vi "Supervisor Read Client.vi"() -> ()   [LabVIEW 2017]
uses:
  <vilib>/OPCUA/controls/NodeIds.ctl
  <vilib>/OPCUA/controls/NodeId.ctl
  <vilib>/OPCUA/NI OPC UA Client.lvlib
panel:
  in  "error in (no error)":errorcluster
  in  "stop":bool
  out "error out":errorcluster
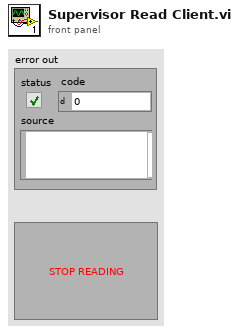
[diagram p1: front panel]
types:
  T1 = cluster{"message mode":enum16{"None", "Sign", "Sign and Encrypt"}, "security":enum16{"Basic256", "Basic128Rsa15"}}
  T2 = typedef "NodeIds.ctl" = T3[]
  T3 = typedef "NodeId.ctl" = string
  T4 = typedef "OPC UA Client Refnum.ctl" = refnum<k21>
  T5 = typedef "Subscription ID.ctl" = u32
  T6 = typedef "Subscription Data Change.ctl" = cluster{"node ID":T3, " value":variant, "timestamp":timestamp, "data type":T7, "status code":T8}
  T7 = typedef "Data Type.ctl" = u16
  T8 = typedef "OPC UA StatusCode.ctl" = u32
  T9 = cluster{"[0]":sgl, "[1]":sgl, "[2]":sgl, "[3]":sgl, "[4]":sgl, "[5]":sgl, "[6]":sgl, "[7]":sgl, "[8]":sgl, "[9]":sgl, "[10]":sgl, "[11]":sgl, "[12]":sgl, "[13]":sgl, "[14]":sgl, "[15]":sgl, "[16]":sgl, "[17]":sgl, "[18]":sgl, "[19]":sgl, "[20]":sgl, "[21]":sgl, "[22]":sgl, "[23]":sgl, "[24]":sgl, "[25]":sgl, "[26]":sgl, "[27]":sgl, "[28]":sgl, "[29]":sgl, "[30]":sgl, "[31]":sgl, "[32]":sgl, "[33]":sgl, "[34]":sgl, "[35]":sgl, "[36]":sgl, "[37]":sgl, "[38]":sgl, "[39]":sgl, "[40]":sgl, "[41]":sgl, "[42]":sgl, "[43]":sgl, "[44]":sgl, "[45]":sgl, "[46]":sgl, "[47]":sgl, "[48]":sgl, "[49]":sgl, "[50]":sgl, "[51]":sgl, "[52]":sgl, "[53]":sgl, "[54]":sgl, "[55]":sgl, "[56]":sgl, "[57]":sgl, "[58]":sgl, "[59]":sgl, "[60]":sgl, "[61]":sgl, "[62]":sgl}
  T10 = cluster{"[0]":sgl, "[1]":sgl, "[2]":sgl, "[3]":sgl, "[4]":sgl, "[5]":sgl, "[6]":sgl, "[7]":sgl, "[8]":sgl, "[9]":sgl}
  T11 = cluster{"[0]":bool, "[1]":bool, "[2]":bool, "[3]":bool, "[4]":bool, "[5]":bool, "[6]":bool}
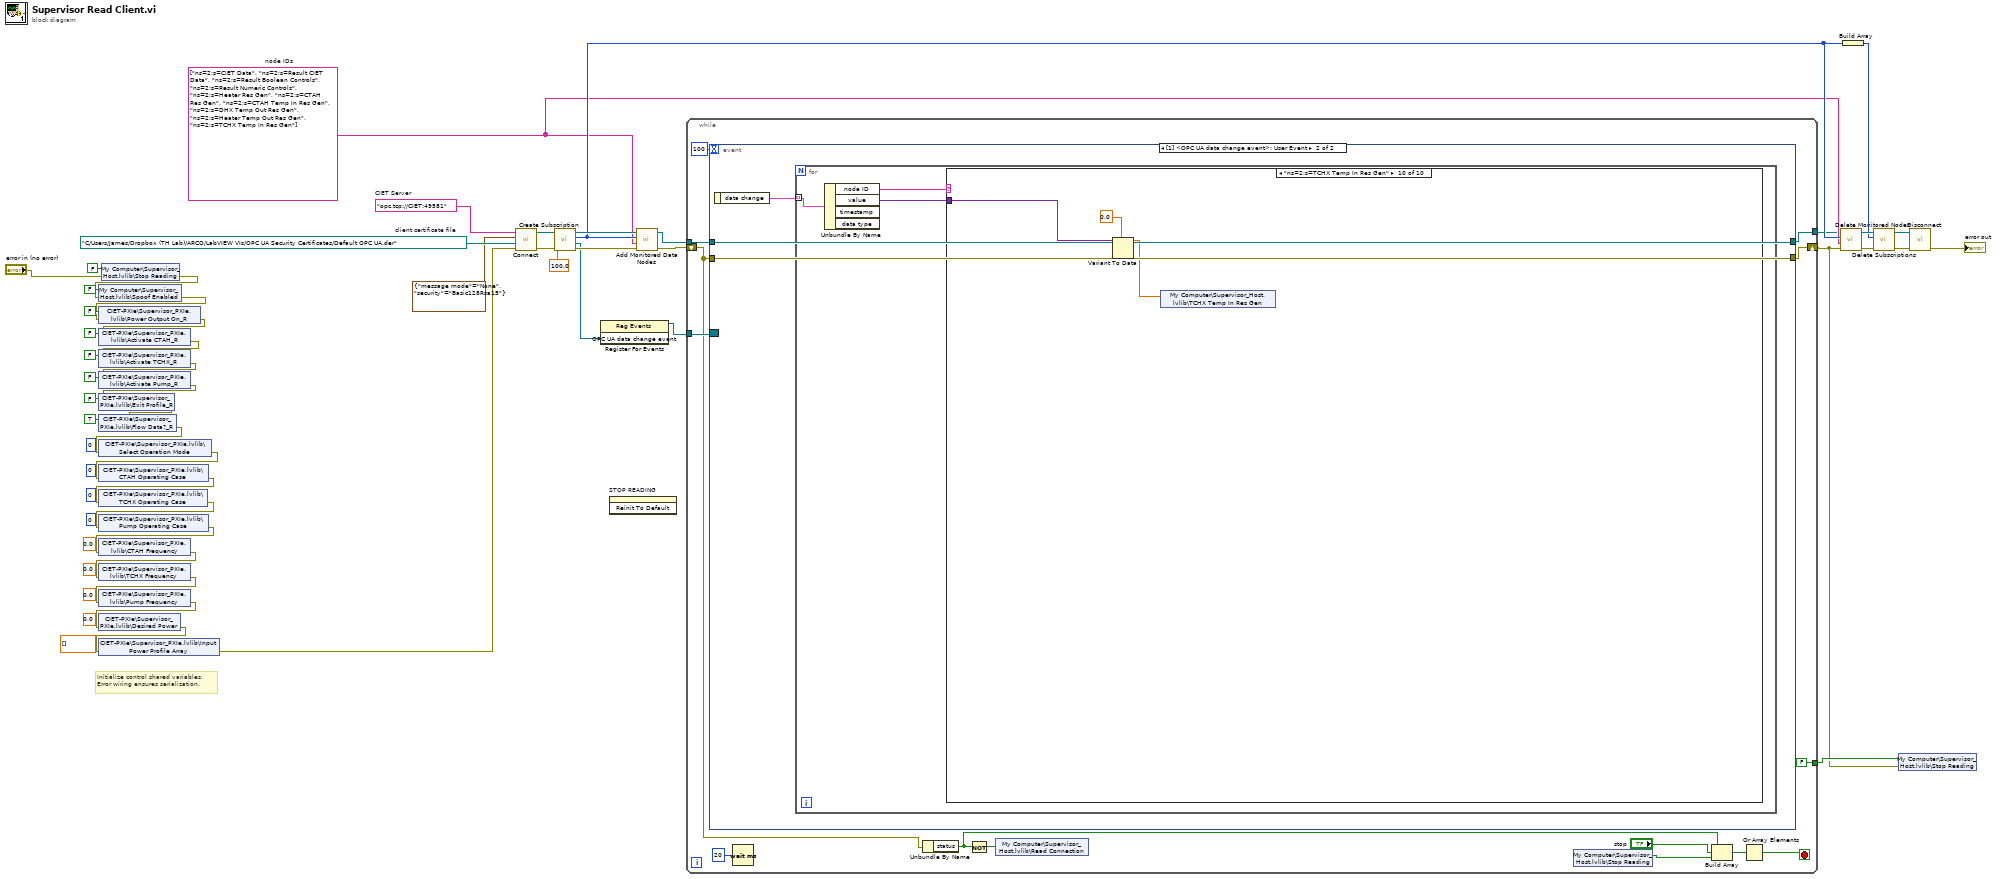
[diagram p0: block diagram]
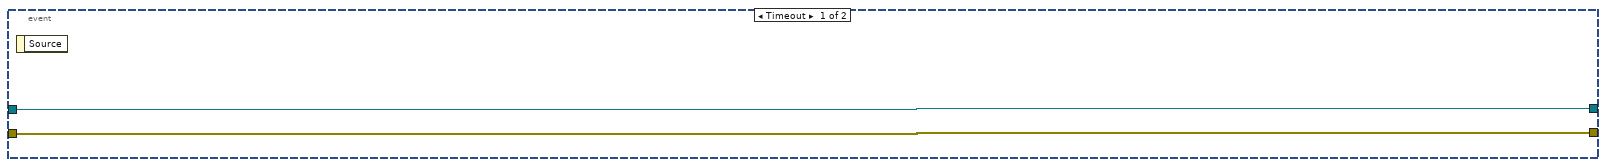
[diagram p2: hidden frame]
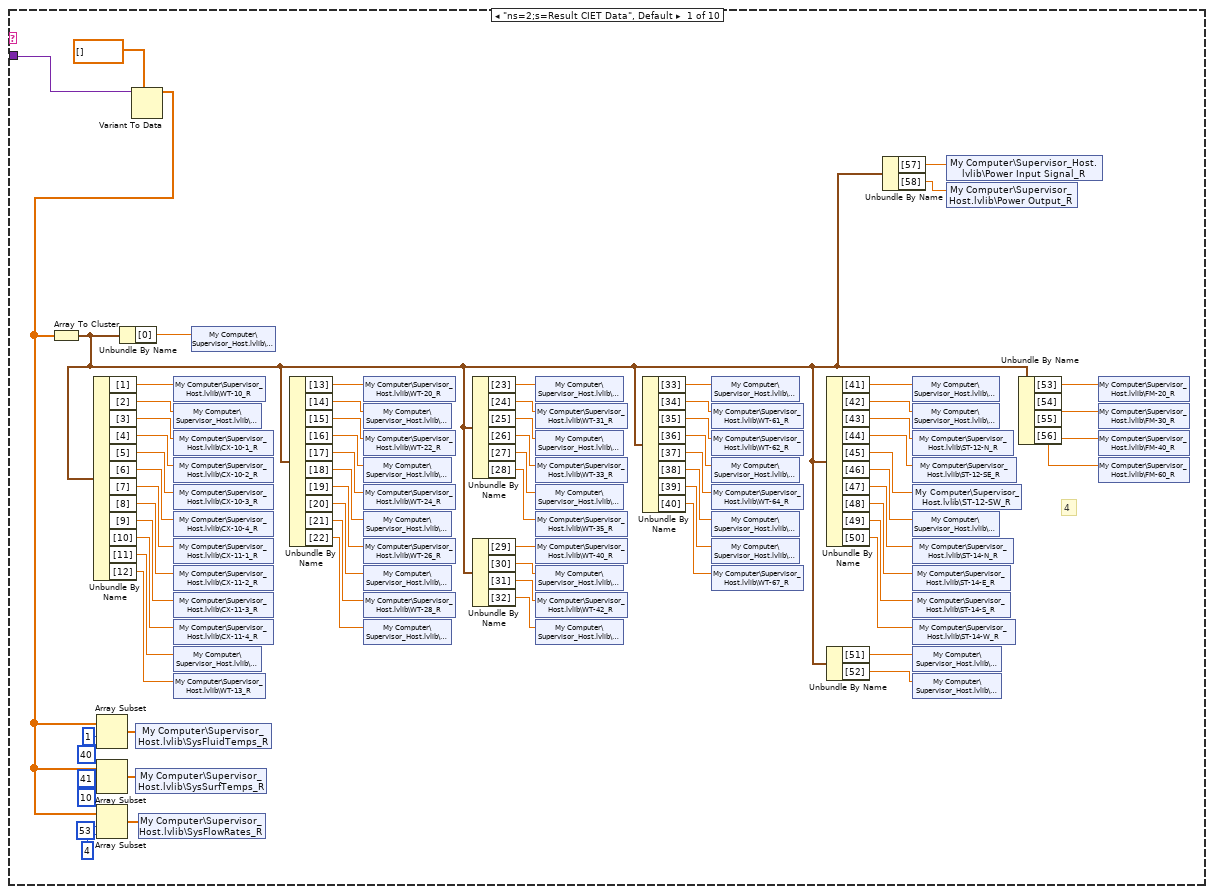
[diagram p3: hidden frame]
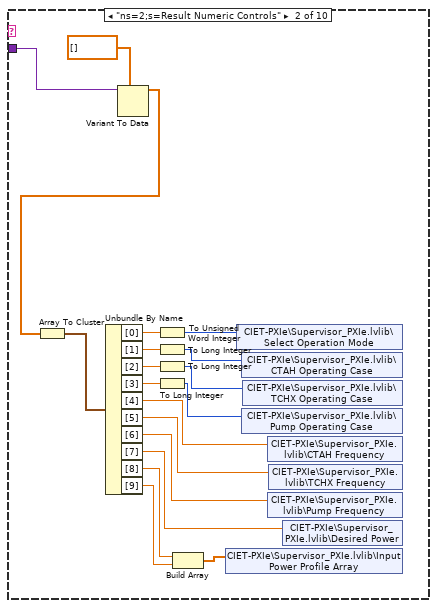
[diagram p4: hidden frame]
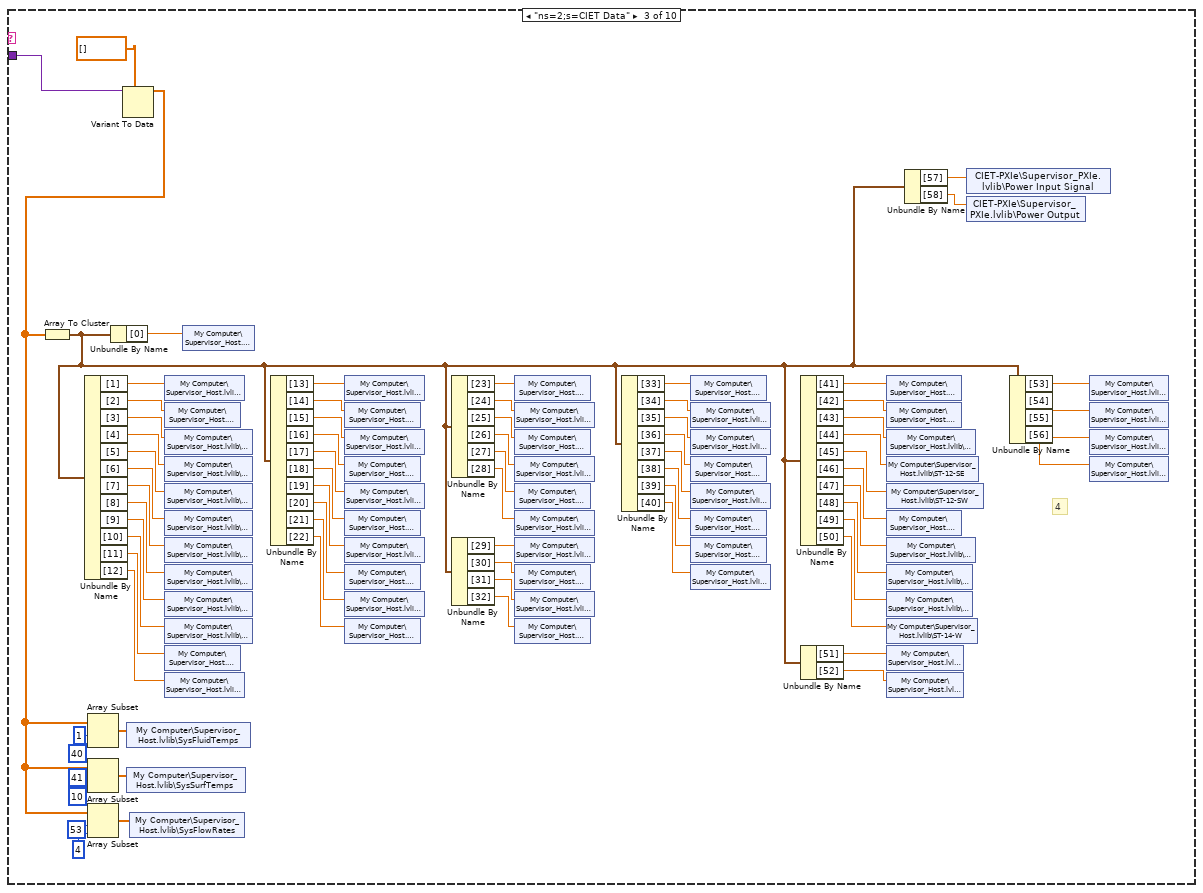
[diagram p5: hidden frame]
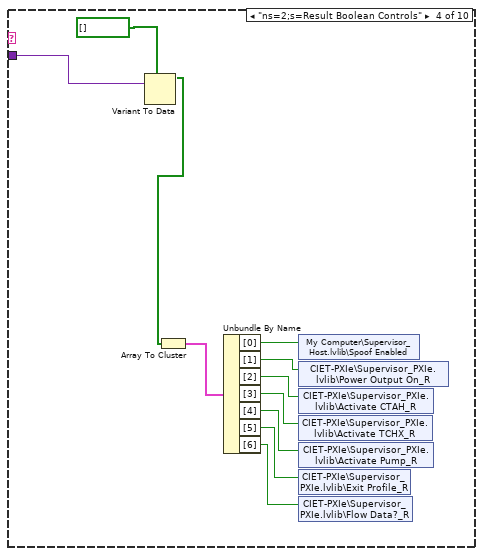
[diagram p6: hidden frame]
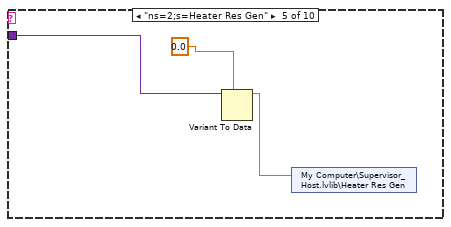
[diagram p7: hidden frame]
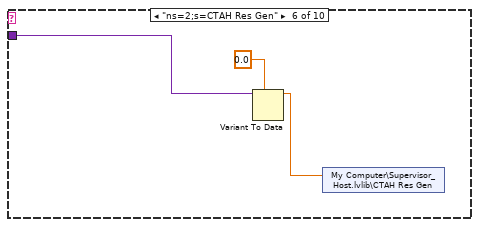
[diagram p8: hidden frame]
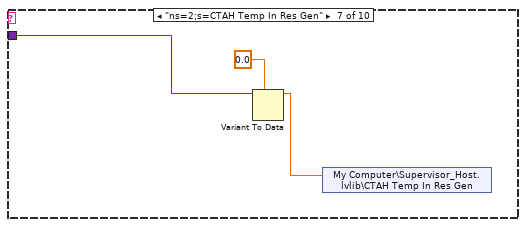
[diagram p9: hidden frame]
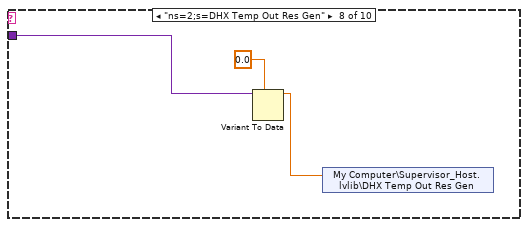
[diagram p10: hidden frame]
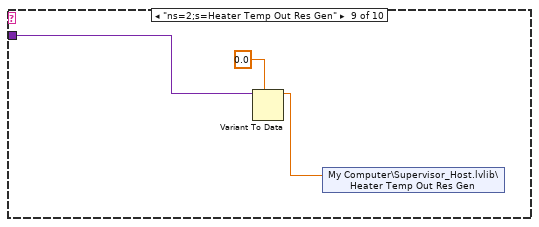
[diagram p11: hidden frame]
diagram:
  w41 = T2 ["ns=2;s=CIET Data", "ns=2;s=Result CIET Data", "ns=2;s=Result Boolean Controls", "ns=2;s=Result Numeric Controls", "ns=2;s=Heater Res Gen", "ns=2;s=CTAH Res Gen", "ns=2;s=CTAH Temp In Res Gen", "ns=2;s=DHX Temp Out Res Gen", "ns=2;s=Heater Temp Out Res Gen", "ns=2;s=TCHX Temp In Res Gen"]  # node IDs
  w56 = path "C:/Users/James/Dropbox (TH Lab)/ARCO/LabVIEW VIs/OPC UA Security Certificates/Default OPC UA.der"  # client certificate file
  w57 = "opc.tcp://CIET:49581"  # CIET Server
  # "Initialize control shared variables.\nError wiring ensures serialization."
  n1 = shared-variable "My Computer\\Supervisor_Host.lvlib\\Stop Reading"(FALSE ("Stop Reading"), error in="error in (no error)") -> (error out=w3:errorcluster)
  n2 = shared-variable "My Computer\\Supervisor_Host.lvlib\\Spoof Enabled"(FALSE ("Spoof Enabled"), error in=w3) -> (error out=w29:errorcluster)
  n3 = shared-variable "CIET-PXIe\\Supervisor_PXIe.lvlib\\Power Output On_R"(FALSE ("Power Output On_R"), error in=w29) -> (error out=w28:errorcluster)
  n4 = shared-variable "CIET-PXIe\\Supervisor_PXIe.lvlib\\Activate CTAH_R"(FALSE ("Activate CTAH_R"), error in=w28) -> (error out=w27:errorcluster)
  n5 = shared-variable "CIET-PXIe\\Supervisor_PXIe.lvlib\\Activate TCHX_R"(FALSE ("Activate TCHX_R"), error in=w27) -> (error out=w26:errorcluster)
  n6 = shared-variable "CIET-PXIe\\Supervisor_PXIe.lvlib\\Activate Pump_R"(FALSE ("Activate Pump_R"), error in=w26) -> (error out=w25:errorcluster)
  n7 = shared-variable "CIET-PXIe\\Supervisor_PXIe.lvlib\\Exit Profile_R"(FALSE ("Exit Profile_R"), error in=w25) -> (error out=w24:errorcluster)
  n8 = shared-variable "CIET-PXIe\\Supervisor_PXIe.lvlib\\Flow Data?_R"(TRUE ("Flow Data?_R"), error in=w24) -> (error out=w23:errorcluster)
  n9 = shared-variable "CIET-PXIe\\Supervisor_PXIe.lvlib\\Select Operation Mode"(u16 0 ("Select Operation Mode"), error in=w23) -> (error out=w22:errorcluster)
  n10 = shared-variable "CIET-PXIe\\Supervisor_PXIe.lvlib\\CTAH Operating Case"(0 ("CTAH Operating Case"), error in=w22) -> (error out=w21:errorcluster)
  n11 = shared-variable "CIET-PXIe\\Supervisor_PXIe.lvlib\\TCHX Operating Case"(0 ("TCHX Operating Case"), error in=w21) -> (error out=w20:errorcluster)
  n12 = shared-variable "CIET-PXIe\\Supervisor_PXIe.lvlib\\Pump Operating Case"(0 ("Pump Operating Case"), error in=w20) -> (error out=w19:errorcluster)
  n13 = shared-variable "CIET-PXIe\\Supervisor_PXIe.lvlib\\CTAH Frequency"(sgl 0.0 ("CTAH Frequency"), error in=w19) -> (error out=w18:errorcluster)
  n14 = shared-variable "CIET-PXIe\\Supervisor_PXIe.lvlib\\TCHX Frequency"(sgl 0.0 ("TCHX Frequency"), error in=w18) -> (error out=w17:errorcluster)
  n15 = shared-variable "CIET-PXIe\\Supervisor_PXIe.lvlib\\Pump Frequency"(sgl 0.0 ("Pump Frequency"), error in=w17) -> (error out=w16:errorcluster)
  n16 = shared-variable "CIET-PXIe\\Supervisor_PXIe.lvlib\\Desired Power"(sgl 0.0 ("Desired Power"), error in=w16) -> (error out=w15:errorcluster)
  n17 = shared-variable "CIET-PXIe\\Supervisor_PXIe.lvlib\\Input Power Profile Array"(dbl[] [] ("Input Power Profile Array"), error in=w15) -> (error out=w14:errorcluster)
  n18 = call <vilib>:"Connect.vi"("error in (no error)"=w14, "client certificate file"=w56, "security policy"=T1 {"message mode"=enum."None", "security"=enum."Basic128Rsa15"}, "server endpoint URL"=w57) -> ("error out"=w37:errorcluster, "OPC UA client refnum out"=w54:T4)  [unwired: 5 in, 1 out]
  n19 = call <vilib>:"Create Subscription.vi"("error in (no error)"=w37, "publishing interval (1000 ms)"=100.0, "OPC UA client refnum in"=w54) -> ("error out"=w52:errorcluster, "OPC UA data change event"=w51:refnum<user-event>, "subscription ID out"=w46:T5, "OPC UA client refnum out"=w53:T4)  [unwired: 4 in, 1 out]
  n20 = register-events(w51) -> (reference out=w44:refnum<event-registration>)  [unwired: 2 in, 1 out]
  n21 = invoke on="STOP READING" class="Bool" method="Reinit To Default"() -> ()  [unwired: 3 in, 3 out]
  n22 = call <vilib>:"Add Monitored Data Nodes.vi"("error in (no error)"=w52, "node IDs"=w41, "subscription ID in"=w46, "OPC UA client refnum in"=w53) -> ("error out"=w42:errorcluster, "OPC UA client refnum out"=w43:T4)  [unwired: 4 in, 2 out]
  n23 = while {
    tunnel: w44 -> [w72]
    tunnel: w43 -> [w71]
    tunnel: [w70] -> w40
    tunnel: [FALSE] -> w38
    shift-right: [w66] -> w1
    shift-left: w42 -> [w65]
    stop <- w64 stop-if-true
    n24 = event shown="[1] <OPC UA data change event>: User Event" {
      selector: w72 -> [_ _]
      dyn-events: _ -> [_ _]
      timeout: 100 -> [_ _]
      tunnel: w71 -> [w74 w77]
      tunnel: [w74 w77] -> w70
      tunnel: w65 -> [w73 w76]
      tunnel: [w73 w76] -> w66
      event Timeout {
        n25 = event-data() -> ()  [unwired: 1 in, 1 out]
      }
      event User Event {
        n26 = event-data() -> ("data change"=w75:T6[])  [unwired: 1 in]
        n27 = for {
          tunnel: w75 -> [w80] mode=indexing
          n28 = Unbundle By Name(w80) -> ("node ID"=w79:T3, "value"=w78:variant)  [unwired: 2 out]
          n29 = case shown="\"ns=2;s=TCHX Temp In Res Gen\"" w79 {
            tunnel: w78 -> [w86 w169 w184 w245 w257 w260 w263 w266 w269 w272]
            frame "ns=2;s=Result CIET Data", Default {
              # "4"
              n30 = Variant To Data(type=sgl[] [], Variant=w86) -> (data=w85:sgl[])  [unwired: 1 in, 1 out]
              n31 = Array To Cluster(array=w85) -> (cluster=w83:T9)
              n32 = Unbundle By Name(w83) -> ("[1]"=w93:sgl, "[2]"=w95:sgl, "[3]"=w96:sgl, "[4]"=w97:sgl, "[5]"=w98:sgl, "[6]"=w99:sgl, "[7]"=w100:sgl, "[8]"=w101:sgl, "[9]"=w102:sgl, "[10]"=w103:sgl, "[11]"=w104:sgl, "[12]"=w105:sgl)
              n33 = Array Subset(array=w85, index=1, length=40) -> (w150:sgl[])
              n34 = Array Subset(array=w85, index=41, length=10) -> (w151:sgl[])
              n35 = Array Subset(array=w85, index=53, length=4) -> (w152:sgl[])
              n36 = Unbundle By Name(w83) -> ("[0]"=w94:sgl)
              n37 = shared-variable "My Computer\\Supervisor_Host.lvlib\\SysFluidTemps_R"(w150) -> ()  [unwired: 1 in, 1 out]
              n38 = shared-variable "My Computer\\Supervisor_Host.lvlib\\SysSurfTemps_R"(w151) -> ()  [unwired: 1 in, 1 out]
              n39 = shared-variable "My Computer\\Supervisor_Host.lvlib\\SysFlowRates_R"(w152) -> ()  [unwired: 1 in, 1 out]
              n40 = shared-variable "My Computer\\Supervisor_Host.lvlib\\WT-10_R"(w93) -> ()  [unwired: 1 in, 1 out]
              n41 = shared-variable "My Computer\\Supervisor_Host.lvlib\\BT-11_R"(w95) -> ()  [unwired: 1 in, 1 out]
              n42 = shared-variable "My Computer\\Supervisor_Host.lvlib\\CX-10-1_R"(w96) -> ()  [unwired: 1 in, 1 out]
              n43 = shared-variable "My Computer\\Supervisor_Host.lvlib\\CX-10-2_R"(w97) -> ()  [unwired: 1 in, 1 out]
              n44 = shared-variable "My Computer\\Supervisor_Host.lvlib\\CX-10-3_R"(w98) -> ()  [unwired: 1 in, 1 out]
              n45 = shared-variable "My Computer\\Supervisor_Host.lvlib\\CX-10-4_R"(w99) -> ()  [unwired: 1 in, 1 out]
              n46 = shared-variable "My Computer\\Supervisor_Host.lvlib\\CX-11-1_R"(w100) -> ()  [unwired: 1 in, 1 out]
              n47 = shared-variable "My Computer\\Supervisor_Host.lvlib\\CX-11-2_R"(w101) -> ()  [unwired: 1 in, 1 out]
              n48 = shared-variable "My Computer\\Supervisor_Host.lvlib\\CX-11-3_R"(w102) -> ()  [unwired: 1 in, 1 out]
              n49 = shared-variable "My Computer\\Supervisor_Host.lvlib\\CX-11-4_R"(w103) -> ()  [unwired: 1 in, 1 out]
              n50 = shared-variable "My Computer\\Supervisor_Host.lvlib\\BT-12_R"(w104) -> ()  [unwired: 1 in, 1 out]
              n51 = shared-variable "My Computer\\Supervisor_Host.lvlib\\WT-13_R"(w105) -> ()  [unwired: 1 in, 1 out]
              n52 = shared-variable "My Computer\\Supervisor_Host.lvlib\\Time_R"(w94) -> ()  [unwired: 1 in, 1 out]
              n53 = Unbundle By Name(w83) -> ("[13]"=w106:sgl, "[14]"=w107:sgl, "[15]"=w108:sgl, "[16]"=w109:sgl, "[17]"=w110:sgl, "[18]"=w111:sgl, "[19]"=w112:sgl, "[20]"=w113:sgl, "[21]"=w114:sgl, "[22]"=w115:sgl)
              n54 = shared-variable "My Computer\\Supervisor_Host.lvlib\\WT-20_R"(w106) -> ()  [unwired: 1 in, 1 out]
              n55 = shared-variable "My Computer\\Supervisor_Host.lvlib\\BT-21_R"(w107) -> ()  [unwired: 1 in, 1 out]
              n56 = shared-variable "My Computer\\Supervisor_Host.lvlib\\WT-22_R"(w108) -> ()  [unwired: 1 in, 1 out]
              n57 = shared-variable "My Computer\\Supervisor_Host.lvlib\\BT-23_R"(w109) -> ()  [unwired: 1 in, 1 out]
              n58 = shared-variable "My Computer\\Supervisor_Host.lvlib\\WT-24_R"(w110) -> ()  [unwired: 1 in, 1 out]
              n59 = shared-variable "My Computer\\Supervisor_Host.lvlib\\BT-25_R"(w111) -> ()  [unwired: 1 in, 1 out]
              n60 = shared-variable "My Computer\\Supervisor_Host.lvlib\\WT-26_R"(w112) -> ()  [unwired: 1 in, 1 out]
              n61 = shared-variable "My Computer\\Supervisor_Host.lvlib\\BT-27_R"(w113) -> ()  [unwired: 1 in, 1 out]
              n62 = shared-variable "My Computer\\Supervisor_Host.lvlib\\WT-28_R"(w114) -> ()  [unwired: 1 in, 1 out]
              n63 = shared-variable "My Computer\\Supervisor_Host.lvlib\\BT-29_R"(w115) -> ()  [unwired: 1 in, 1 out]
              n64 = Unbundle By Name(w83) -> ("[23]"=w116:sgl, "[24]"=w117:sgl, "[25]"=w118:sgl, "[26]"=w119:sgl, "[27]"=w120:sgl, "[28]"=w121:sgl)
              n65 = Unbundle By Name(w83) -> ("[29]"=w122:sgl, "[30]"=w123:sgl, "[31]"=w124:sgl, "[32]"=w125:sgl)
              n66 = shared-variable "My Computer\\Supervisor_Host.lvlib\\BT-30_R"(w116) -> ()  [unwired: 1 in, 1 out]
              n67 = shared-variable "My Computer\\Supervisor_Host.lvlib\\WT-31_R"(w117) -> ()  [unwired: 1 in, 1 out]
              n68 = shared-variable "My Computer\\Supervisor_Host.lvlib\\BT-32_R"(w118) -> ()  [unwired: 1 in, 1 out]
              n69 = shared-variable "My Computer\\Supervisor_Host.lvlib\\WT-33_R"(w119) -> ()  [unwired: 1 in, 1 out]
              n70 = shared-variable "My Computer\\Supervisor_Host.lvlib\\BT-34_R"(w120) -> ()  [unwired: 1 in, 1 out]
              n71 = shared-variable "My Computer\\Supervisor_Host.lvlib\\WT-35_R"(w121) -> ()  [unwired: 1 in, 1 out]
              n72 = shared-variable "My Computer\\Supervisor_Host.lvlib\\WT-40_R"(w122) -> ()  [unwired: 1 in, 1 out]
              n73 = shared-variable "My Computer\\Supervisor_Host.lvlib\\BT-41_R"(w123) -> ()  [unwired: 1 in, 1 out]
              n74 = shared-variable "My Computer\\Supervisor_Host.lvlib\\WT-42_R"(w124) -> ()  [unwired: 1 in, 1 out]
              n75 = shared-variable "My Computer\\Supervisor_Host.lvlib\\BT-43_R"(w125) -> ()  [unwired: 1 in, 1 out]
              n76 = Unbundle By Name(w83) -> ("[33]"=w126:sgl, "[34]"=w127:sgl, "[35]"=w128:sgl, "[36]"=w129:sgl, "[37]"=w130:sgl, "[38]"=w131:sgl, "[39]"=w132:sgl, "[40]"=w133:sgl)
              n77 = shared-variable "My Computer\\Supervisor_Host.lvlib\\BT-60_R"(w126) -> ()  [unwired: 1 in, 1 out]
              n78 = shared-variable "My Computer\\Supervisor_Host.lvlib\\WT-61_R"(w127) -> ()  [unwired: 1 in, 1 out]
              n79 = shared-variable "My Computer\\Supervisor_Host.lvlib\\WT-62_R"(w128) -> ()  [unwired: 1 in, 1 out]
              n80 = shared-variable "My Computer\\Supervisor_Host.lvlib\\BT-63_R"(w129) -> ()  [unwired: 1 in, 1 out]
              n81 = shared-variable "My Computer\\Supervisor_Host.lvlib\\WT-64_R"(w130) -> ()  [unwired: 1 in, 1 out]
              n82 = shared-variable "My Computer\\Supervisor_Host.lvlib\\BT-65_R"(w131) -> ()  [unwired: 1 in, 1 out]
              n83 = shared-variable "My Computer\\Supervisor_Host.lvlib\\BT-66_R"(w132) -> ()  [unwired: 1 in, 1 out]
              n84 = shared-variable "My Computer\\Supervisor_Host.lvlib\\WT-67_R"(w133) -> ()  [unwired: 1 in, 1 out]
              n85 = Unbundle By Name(w83) -> ("[41]"=w134:sgl, "[42]"=w135:sgl, "[43]"=w136:sgl, "[44]"=w137:sgl, "[45]"=w138:sgl, "[46]"=w139:sgl, "[47]"=w140:sgl, "[48]"=w141:sgl, "[49]"=w142:sgl, "[50]"=w143:sgl)
              n86 = Unbundle By Name(w83) -> ("[51]"=w144:sgl, "[52]"=w145:sgl)
              n87 = Unbundle By Name(w83) -> ("[57]"=w82:sgl, "[58]"=w81:sgl)
              n88 = shared-variable "My Computer\\Supervisor_Host.lvlib\\ST-10_R"(w134) -> ()  [unwired: 1 in, 1 out]
              n89 = shared-variable "My Computer\\Supervisor_Host.lvlib\\ST-11_R"(w135) -> ()  [unwired: 1 in, 1 out]
              n90 = shared-variable "My Computer\\Supervisor_Host.lvlib\\ST-12-N_R"(w136) -> ()  [unwired: 1 in, 1 out]
              n91 = shared-variable "My Computer\\Supervisor_Host.lvlib\\ST-12-SE_R"(w137) -> ()  [unwired: 1 in, 1 out]
              n92 = shared-variable "My Computer\\Supervisor_Host.lvlib\\ST-12-SW_R"(w138) -> ()  [unwired: 1 in, 1 out]
              n93 = shared-variable "My Computer\\Supervisor_Host.lvlib\\ST-13_R"(w139) -> ()  [unwired: 1 in, 1 out]
              n94 = shared-variable "My Computer\\Supervisor_Host.lvlib\\ST-14-N_R"(w140) -> ()  [unwired: 1 in, 1 out]
              n95 = shared-variable "My Computer\\Supervisor_Host.lvlib\\ST-14-E_R"(w141) -> ()  [unwired: 1 in, 1 out]
              n96 = shared-variable "My Computer\\Supervisor_Host.lvlib\\ST-14-S_R"(w142) -> ()  [unwired: 1 in, 1 out]
              n97 = shared-variable "My Computer\\Supervisor_Host.lvlib\\ST-14-W_R"(w143) -> ()  [unwired: 1 in, 1 out]
              n98 = shared-variable "My Computer\\Supervisor_Host.lvlib\\AT-01_R"(w144) -> ()  [unwired: 1 in, 1 out]
              n99 = shared-variable "My Computer\\Supervisor_Host.lvlib\\AT-02_R"(w145) -> ()  [unwired: 1 in, 1 out]
              n100 = shared-variable "My Computer\\Supervisor_Host.lvlib\\Power Input Signal_R"(w82) -> ()  [unwired: 1 in, 1 out]
              n101 = shared-variable "My Computer\\Supervisor_Host.lvlib\\Power Output_R"(w81) -> ()  [unwired: 1 in, 1 out]
              n102 = Unbundle By Name(w83) -> ("[53]"=w146:sgl, "[54]"=w147:sgl, "[55]"=w148:sgl, "[56]"=w149:sgl)
              n103 = shared-variable "My Computer\\Supervisor_Host.lvlib\\FM-20_R"(w146) -> ()  [unwired: 1 in, 1 out]
              n104 = shared-variable "My Computer\\Supervisor_Host.lvlib\\FM-30_R"(w147) -> ()  [unwired: 1 in, 1 out]
              n105 = shared-variable "My Computer\\Supervisor_Host.lvlib\\FM-40_R"(w148) -> ()  [unwired: 1 in, 1 out]
              n106 = shared-variable "My Computer\\Supervisor_Host.lvlib\\FM-60_R"(w149) -> ()  [unwired: 1 in, 1 out]
            }
            frame "ns=2;s=Result Numeric Controls" {
              n107 = Variant To Data(type=sgl[] [], Variant=w169) -> (data=w171:sgl[])  [unwired: 1 in, 1 out]
              n108 = Array To Cluster(array=w171) -> (cluster=w170:T10)
              n109 = Unbundle By Name(w170) -> ("[0]"=w167:sgl, "[1]"=w166:sgl, "[2]"=w165:sgl, "[3]"=w164:sgl, "[4]"=w159:sgl, "[5]"=w158:sgl, "[6]"=w157:sgl, "[7]"=w156:sgl, "[8]"=w154:sgl, "[9]"=w153:sgl)
              n110 = To Unsigned Word Integer(number=w167) -> (unsigned 16bit integer=w163:u16)
              n111 = To Long Integer(number=w166) -> (32bit integer=w162:i32)
              n112 = To Long Integer(number=w165) -> (32bit integer=w161:i32)
              n113 = To Long Integer(number=w164) -> (32bit integer=w160:i32)
              n114 = Build Array(w154, w153) -> (w155:sgl[])
              n115 = shared-variable "CIET-PXIe\\Supervisor_PXIe.lvlib\\Input Power Profile Array"(w155) -> ()  [unwired: 1 in, 1 out]
              n116 = shared-variable "CIET-PXIe\\Supervisor_PXIe.lvlib\\Select Operation Mode"(w163) -> ()  [unwired: 1 in, 1 out]
              n117 = shared-variable "CIET-PXIe\\Supervisor_PXIe.lvlib\\CTAH Operating Case"(w162) -> ()  [unwired: 1 in, 1 out]
              n118 = shared-variable "CIET-PXIe\\Supervisor_PXIe.lvlib\\Pump Operating Case"(w160) -> ()  [unwired: 1 in, 1 out]
              n119 = shared-variable "CIET-PXIe\\Supervisor_PXIe.lvlib\\TCHX Operating Case"(w161) -> ()  [unwired: 1 in, 1 out]
              n120 = shared-variable "CIET-PXIe\\Supervisor_PXIe.lvlib\\CTAH Frequency"(w159) -> ()  [unwired: 1 in, 1 out]
              n121 = shared-variable "CIET-PXIe\\Supervisor_PXIe.lvlib\\Pump Frequency"(w157) -> ()  [unwired: 1 in, 1 out]
              n122 = shared-variable "CIET-PXIe\\Supervisor_PXIe.lvlib\\TCHX Frequency"(w158) -> ()  [unwired: 1 in, 1 out]
              n123 = shared-variable "CIET-PXIe\\Supervisor_PXIe.lvlib\\Desired Power"(w156) -> ()  [unwired: 1 in, 1 out]
            }
            frame "ns=2;s=CIET Data" {
              # "4"
              n124 = Variant To Data(type=sgl[] [], Variant=w184) -> (data=w181:sgl[])  [unwired: 1 in, 1 out]
              n125 = Array To Cluster(array=w181) -> (cluster=w174:T9)
              n126 = Unbundle By Name(w174) -> ("[1]"=w183:sgl, "[2]"=w186:sgl, "[3]"=w187:sgl, "[4]"=w188:sgl, "[5]"=w189:sgl, "[6]"=w190:sgl, "[7]"=w191:sgl, "[8]"=w192:sgl, "[9]"=w193:sgl, "[10]"=w194:sgl, "[11]"=w195:sgl, "[12]"=w196:sgl)
              n127 = Array Subset(array=w181, index=1, length=40) -> (w241:sgl[])
              n128 = Array Subset(array=w181, index=41, length=10) -> (w242:sgl[])
              n129 = Array Subset(array=w181, index=53, length=4) -> (w243:sgl[])
              n130 = Unbundle By Name(w174) -> ("[0]"=w185:sgl)
              n131 = shared-variable "My Computer\\Supervisor_Host.lvlib\\SysFluidTemps"(w241) -> ()  [unwired: 1 in, 1 out]
              n132 = shared-variable "My Computer\\Supervisor_Host.lvlib\\SysSurfTemps"(w242) -> ()  [unwired: 1 in, 1 out]
              n133 = shared-variable "My Computer\\Supervisor_Host.lvlib\\SysFlowRates"(w243) -> ()  [unwired: 1 in, 1 out]
              n134 = shared-variable "My Computer\\Supervisor_Host.lvlib\\WT-10"(w183) -> ()  [unwired: 1 in, 1 out]
              n135 = shared-variable "My Computer\\Supervisor_Host.lvlib\\BT-11"(w186) -> ()  [unwired: 1 in, 1 out]
              n136 = shared-variable "My Computer\\Supervisor_Host.lvlib\\CX-10-1"(w187) -> ()  [unwired: 1 in, 1 out]
              n137 = shared-variable "My Computer\\Supervisor_Host.lvlib\\CX-10-2"(w188) -> ()  [unwired: 1 in, 1 out]
              n138 = shared-variable "My Computer\\Supervisor_Host.lvlib\\CX-10-3"(w189) -> ()  [unwired: 1 in, 1 out]
              n139 = shared-variable "My Computer\\Supervisor_Host.lvlib\\CX-10-4"(w190) -> ()  [unwired: 1 in, 1 out]
              n140 = shared-variable "My Computer\\Supervisor_Host.lvlib\\CX-11-1"(w191) -> ()  [unwired: 1 in, 1 out]
              n141 = shared-variable "My Computer\\Supervisor_Host.lvlib\\CX-11-2"(w192) -> ()  [unwired: 1 in, 1 out]
              n142 = shared-variable "My Computer\\Supervisor_Host.lvlib\\CX-11-3"(w193) -> ()  [unwired: 1 in, 1 out]
              n143 = shared-variable "My Computer\\Supervisor_Host.lvlib\\CX-11-4"(w194) -> ()  [unwired: 1 in, 1 out]
              n144 = shared-variable "My Computer\\Supervisor_Host.lvlib\\BT-12"(w195) -> ()  [unwired: 1 in, 1 out]
              n145 = shared-variable "My Computer\\Supervisor_Host.lvlib\\WT-13"(w196) -> ()  [unwired: 1 in, 1 out]
              n146 = shared-variable "My Computer\\Supervisor_Host.lvlib\\Time"(w185) -> ()  [unwired: 1 in, 1 out]
              n147 = Unbundle By Name(w174) -> ("[13]"=w197:sgl, "[14]"=w198:sgl, "[15]"=w199:sgl, "[16]"=w200:sgl, "[17]"=w201:sgl, "[18]"=w202:sgl, "[19]"=w203:sgl, "[20]"=w204:sgl, "[21]"=w205:sgl, "[22]"=w206:sgl)
              n148 = shared-variable "My Computer\\Supervisor_Host.lvlib\\WT-20"(w197) -> ()  [unwired: 1 in, 1 out]
              n149 = shared-variable "My Computer\\Supervisor_Host.lvlib\\BT-21"(w198) -> ()  [unwired: 1 in, 1 out]
              n150 = shared-variable "My Computer\\Supervisor_Host.lvlib\\WT-22"(w199) -> ()  [unwired: 1 in, 1 out]
              n151 = shared-variable "My Computer\\Supervisor_Host.lvlib\\BT-23"(w200) -> ()  [unwired: 1 in, 1 out]
              n152 = shared-variable "My Computer\\Supervisor_Host.lvlib\\WT-24"(w201) -> ()  [unwired: 1 in, 1 out]
              n153 = shared-variable "My Computer\\Supervisor_Host.lvlib\\BT-25"(w202) -> ()  [unwired: 1 in, 1 out]
              n154 = shared-variable "My Computer\\Supervisor_Host.lvlib\\WT-26"(w203) -> ()  [unwired: 1 in, 1 out]
              n155 = shared-variable "My Computer\\Supervisor_Host.lvlib\\BT-27"(w204) -> ()  [unwired: 1 in, 1 out]
              n156 = shared-variable "My Computer\\Supervisor_Host.lvlib\\WT-28"(w205) -> ()  [unwired: 1 in, 1 out]
              n157 = shared-variable "My Computer\\Supervisor_Host.lvlib\\BT-29"(w206) -> ()  [unwired: 1 in, 1 out]
              n158 = Unbundle By Name(w174) -> ("[23]"=w207:sgl, "[24]"=w208:sgl, "[25]"=w209:sgl, "[26]"=w210:sgl, "[27]"=w211:sgl, "[28]"=w212:sgl)
              n159 = Unbundle By Name(w174) -> ("[29]"=w213:sgl, "[30]"=w214:sgl, "[31]"=w215:sgl, "[32]"=w216:sgl)
              n160 = shared-variable "My Computer\\Supervisor_Host.lvlib\\BT-30"(w207) -> ()  [unwired: 1 in, 1 out]
              n161 = shared-variable "My Computer\\Supervisor_Host.lvlib\\WT-31"(w208) -> ()  [unwired: 1 in, 1 out]
              n162 = shared-variable "My Computer\\Supervisor_Host.lvlib\\BT-32"(w209) -> ()  [unwired: 1 in, 1 out]
              n163 = shared-variable "My Computer\\Supervisor_Host.lvlib\\WT-33"(w210) -> ()  [unwired: 1 in, 1 out]
              n164 = shared-variable "My Computer\\Supervisor_Host.lvlib\\BT-34"(w211) -> ()  [unwired: 1 in, 1 out]
              n165 = shared-variable "My Computer\\Supervisor_Host.lvlib\\WT-35"(w212) -> ()  [unwired: 1 in, 1 out]
              n166 = shared-variable "My Computer\\Supervisor_Host.lvlib\\WT-40"(w213) -> ()  [unwired: 1 in, 1 out]
              n167 = shared-variable "My Computer\\Supervisor_Host.lvlib\\BT-41"(w214) -> ()  [unwired: 1 in, 1 out]
              n168 = shared-variable "My Computer\\Supervisor_Host.lvlib\\WT-42"(w215) -> ()  [unwired: 1 in, 1 out]
              n169 = shared-variable "My Computer\\Supervisor_Host.lvlib\\BT-43"(w216) -> ()  [unwired: 1 in, 1 out]
              n170 = Unbundle By Name(w174) -> ("[33]"=w217:sgl, "[34]"=w218:sgl, "[35]"=w219:sgl, "[36]"=w220:sgl, "[37]"=w221:sgl, "[38]"=w222:sgl, "[39]"=w223:sgl, "[40]"=w224:sgl)
              n171 = shared-variable "My Computer\\Supervisor_Host.lvlib\\BT-60"(w217) -> ()  [unwired: 1 in, 1 out]
              n172 = shared-variable "My Computer\\Supervisor_Host.lvlib\\WT-61"(w218) -> ()  [unwired: 1 in, 1 out]
              n173 = shared-variable "My Computer\\Supervisor_Host.lvlib\\WT-62"(w219) -> ()  [unwired: 1 in, 1 out]
              n174 = shared-variable "My Computer\\Supervisor_Host.lvlib\\BT-63"(w220) -> ()  [unwired: 1 in, 1 out]
              n175 = shared-variable "My Computer\\Supervisor_Host.lvlib\\WT-64"(w221) -> ()  [unwired: 1 in, 1 out]
              n176 = shared-variable "My Computer\\Supervisor_Host.lvlib\\BT-65"(w222) -> ()  [unwired: 1 in, 1 out]
              n177 = shared-variable "My Computer\\Supervisor_Host.lvlib\\BT-66"(w223) -> ()  [unwired: 1 in, 1 out]
              n178 = shared-variable "My Computer\\Supervisor_Host.lvlib\\WT-67"(w224) -> ()  [unwired: 1 in, 1 out]
              n179 = Unbundle By Name(w174) -> ("[41]"=w225:sgl, "[42]"=w226:sgl, "[43]"=w227:sgl, "[44]"=w228:sgl, "[45]"=w229:sgl, "[46]"=w230:sgl, "[47]"=w231:sgl, "[48]"=w232:sgl, "[49]"=w233:sgl, "[50]"=w234:sgl)
              n180 = Unbundle By Name(w174) -> ("[51]"=w235:sgl, "[52]"=w236:sgl)
              n181 = shared-variable "My Computer\\Supervisor_Host.lvlib\\ST-10"(w225) -> ()  [unwired: 1 in, 1 out]
              n182 = shared-variable "My Computer\\Supervisor_Host.lvlib\\ST-11"(w226) -> ()  [unwired: 1 in, 1 out]
              n183 = shared-variable "My Computer\\Supervisor_Host.lvlib\\ST-12-N"(w227) -> ()  [unwired: 1 in, 1 out]
              n184 = shared-variable "My Computer\\Supervisor_Host.lvlib\\ST-12-SE"(w228) -> ()  [unwired: 1 in, 1 out]
              n185 = shared-variable "My Computer\\Supervisor_Host.lvlib\\ST-12-SW"(w229) -> ()  [unwired: 1 in, 1 out]
              n186 = shared-variable "My Computer\\Supervisor_Host.lvlib\\ST-13"(w230) -> ()  [unwired: 1 in, 1 out]
              n187 = shared-variable "My Computer\\Supervisor_Host.lvlib\\ST-14-N"(w231) -> ()  [unwired: 1 in, 1 out]
              n188 = shared-variable "My Computer\\Supervisor_Host.lvlib\\ST-14-E"(w232) -> ()  [unwired: 1 in, 1 out]
              n189 = shared-variable "My Computer\\Supervisor_Host.lvlib\\ST-14-S"(w233) -> ()  [unwired: 1 in, 1 out]
              n190 = shared-variable "My Computer\\Supervisor_Host.lvlib\\ST-14-W"(w234) -> ()  [unwired: 1 in, 1 out]
              n191 = shared-variable "My Computer\\Supervisor_Host.lvlib\\AT-01"(w235) -> ()  [unwired: 1 in, 1 out]
              n192 = shared-variable "My Computer\\Supervisor_Host.lvlib\\AT-02"(w236) -> ()  [unwired: 1 in, 1 out]
              n193 = Unbundle By Name(w174) -> ("[57]"=w173:sgl, "[58]"=w172:sgl)
              n194 = shared-variable "CIET-PXIe\\Supervisor_PXIe.lvlib\\Power Input Signal"(w173) -> ()  [unwired: 1 in, 1 out]
              n195 = shared-variable "CIET-PXIe\\Supervisor_PXIe.lvlib\\Power Output"(w172) -> ()  [unwired: 1 in, 1 out]
              n196 = Unbundle By Name(w174) -> ("[53]"=w237:sgl, "[54]"=w238:sgl, "[55]"=w239:sgl, "[56]"=w240:sgl)
              n197 = shared-variable "My Computer\\Supervisor_Host.lvlib\\FM-20"(w237) -> ()  [unwired: 1 in, 1 out]
              n198 = shared-variable "My Computer\\Supervisor_Host.lvlib\\FM-30"(w238) -> ()  [unwired: 1 in, 1 out]
              n199 = shared-variable "My Computer\\Supervisor_Host.lvlib\\FM-40"(w239) -> ()  [unwired: 1 in, 1 out]
              n200 = shared-variable "My Computer\\Supervisor_Host.lvlib\\FM-60"(w240) -> ()  [unwired: 1 in, 1 out]
            }
            frame "ns=2;s=Result Boolean Controls" {
              n201 = Variant To Data(type=bool[] [], Variant=w245) -> (data=w244:bool[])  [unwired: 1 in, 1 out]
              n202 = Array To Cluster(array=w244) -> (cluster=w254:T11)
              n203 = Unbundle By Name(w254) -> ("[0]"=w253:bool, "[1]"=w252:bool, "[2]"=w251:bool, "[3]"=w250:bool, "[4]"=w249:bool, "[5]"=w248:bool, "[6]"=w247:bool)
              n204 = shared-variable "My Computer\\Supervisor_Host.lvlib\\Spoof Enabled"(w253) -> ()  [unwired: 1 in, 1 out]
              n205 = shared-variable "CIET-PXIe\\Supervisor_PXIe.lvlib\\Power Output On_R"(w252) -> ()  [unwired: 1 in, 1 out]
              n206 = shared-variable "CIET-PXIe\\Supervisor_PXIe.lvlib\\Activate CTAH_R"(w251) -> ()  [unwired: 1 in, 1 out]
              n207 = shared-variable "CIET-PXIe\\Supervisor_PXIe.lvlib\\Activate TCHX_R"(w250) -> ()  [unwired: 1 in, 1 out]
              n208 = shared-variable "CIET-PXIe\\Supervisor_PXIe.lvlib\\Activate Pump_R"(w249) -> ()  [unwired: 1 in, 1 out]
              n209 = shared-variable "CIET-PXIe\\Supervisor_PXIe.lvlib\\Exit Profile_R"(w248) -> ()  [unwired: 1 in, 1 out]
              n210 = shared-variable "CIET-PXIe\\Supervisor_PXIe.lvlib\\Flow Data?_R"(w247) -> ()  [unwired: 1 in, 1 out]
            }
            frame "ns=2;s=Heater Res Gen" {
              n211 = Variant To Data(type=0.0, Variant=w257) -> (data=w255:dbl)  [unwired: 1 in, 1 out]
              n212 = shared-variable "My Computer\\Supervisor_Host.lvlib\\Heater Res Gen"(w255) -> ()  [unwired: 1 in, 1 out]
            }
            frame "ns=2;s=CTAH Res Gen" {
              n213 = Variant To Data(type=0.0, Variant=w260) -> (data=w258:dbl)  [unwired: 1 in, 1 out]
              n214 = shared-variable "My Computer\\Supervisor_Host.lvlib\\CTAH Res Gen"(w258) -> ()  [unwired: 1 in, 1 out]
            }
            frame "ns=2;s=CTAH Temp In Res Gen" {
              n215 = Variant To Data(type=0.0, Variant=w263) -> (data=w261:dbl)  [unwired: 1 in, 1 out]
              n216 = shared-variable "My Computer\\Supervisor_Host.lvlib\\CTAH Temp In Res Gen"(w261) -> ()  [unwired: 1 in, 1 out]
            }
            frame "ns=2;s=DHX Temp Out Res Gen" {
              n217 = Variant To Data(type=0.0, Variant=w266) -> (data=w264:dbl)  [unwired: 1 in, 1 out]
              n218 = shared-variable "My Computer\\Supervisor_Host.lvlib\\DHX Temp Out Res Gen"(w264) -> ()  [unwired: 1 in, 1 out]
            }
            frame "ns=2;s=Heater Temp Out Res Gen" {
              n219 = Variant To Data(type=0.0, Variant=w269) -> (data=w267:dbl)  [unwired: 1 in, 1 out]
              n220 = shared-variable "My Computer\\Supervisor_Host.lvlib\\Heater Temp Out Res Gen"(w267) -> ()  [unwired: 1 in, 1 out]
            }
            frame "ns=2;s=TCHX Temp In Res Gen" {
              n221 = Variant To Data(type=0.0, Variant=w272) -> (data=w270:dbl)  [unwired: 1 in, 1 out]
              n222 = shared-variable "My Computer\\Supervisor_Host.lvlib\\TCHX Temp In Res Gen"(w270) -> ()  [unwired: 1 in, 1 out]
            }
          }
        }
      }
    }
    n223 = Wait (ms)(milliseconds to wait=u32 20 ("millisecond timer value")) -> ()  [unwired: 1 out]
    n224 = Unbundle By Name(w65) -> ("status"=w60:bool)
    n225 = Not(x=w60) -> (.not. x?=w67:bool)
    n226 = shared-variable "My Computer\\Supervisor_Host.lvlib\\Read Connection"(w67) -> ()  [unwired: 1 in, 1 out]
    n227 = shared-variable "My Computer\\Supervisor_Host.lvlib\\Stop Reading"() -> (w63:bool)  [unwired: 1 in, 1 out]
    n228 = Build Array(w60, "stop", w63) -> (w61:bool[])
    n229 = Or Array Elements(Boolean array=w61) -> (logical OR=w64:bool)
  }
  n230 = call <vilib>:"Delete Monitored Nodes.vi"("error in (no error)"=w1, "node IDs"=w41, "subscription ID in"=w46, "OPC UA client refnum in"=w40) -> ("error out"=w47:errorcluster, "OPC UA client refnum out"=w48:T4)  [unwired: 3 in, 3 out]
  n231 = Build Array(w46) -> (w45:T5[])
  n232 = call <vilib>:"Delete Subscriptions.vi"("error in (no error)"=w47, "subscription IDs"=w45, "OPC UA client refnum in"=w48) -> ("error out"=w49:errorcluster, "OPC UA client refnum out"=w50:T4)  [unwired: 6 in, 1 out]
  n233 = shared-variable "My Computer\\Supervisor_Host.lvlib\\Stop Reading"(w38, error in=w1) -> ()  [unwired: 1 out]
  n234 = call <vilib>:"Disconnect.vi"("error in (no error)"=w49, "OPC UA client refnum in"=w50) -> ("error out"=→"error out":errorcluster)  [unwired: 9 in]
